vi "VoltageScan_easy.vi"() -> ()   [LabVIEW 2016]
uses:
  Input_parameters.ctl
  Dynamic_data.ctl
panel:
  out "Single channel":cluster{"X":dbl[], "Y":dbl[]}[](graph) caption="XY Graph"
  out "Voltages":cluster{"X":dbl[], "Y":dbl[]}[](graph) caption="XY Graph"
  out "Channels":cluster{i32[], dbl[]}[](graph) caption="XY Graph"
  out "Current channel":dbl format="%#_13g"
  out "Current voltage (V)":dbl format="%#_13g"
  in  "Stop":bool
  in  "Input parameters":T1={"Measurement type"=enum."Test", "Sensor type"=enum."One channel", "Input file"="", "Output file"="test.txt", "Open after execution?"=FALSE, "Display channel"=0, "Voltage Delay (s)"=0.5, "Switch Delay (s)"=0.01, "VISA resource name source"="", "VISA resource name LCR"="", "Voltage Limit (V)"=1000.0, "Enable Voltage Auto Range (T:Enable)"=TRUE, "Voltage Manual Range (1.0)"=1.0, "Compliance  Level (uA)"=10.0} {"Voltage Limit (V)" format="%#_13g"; "Voltage Delay (s)" format="%#_13g"; "Switch Delay (s)" format="%#_13g"}
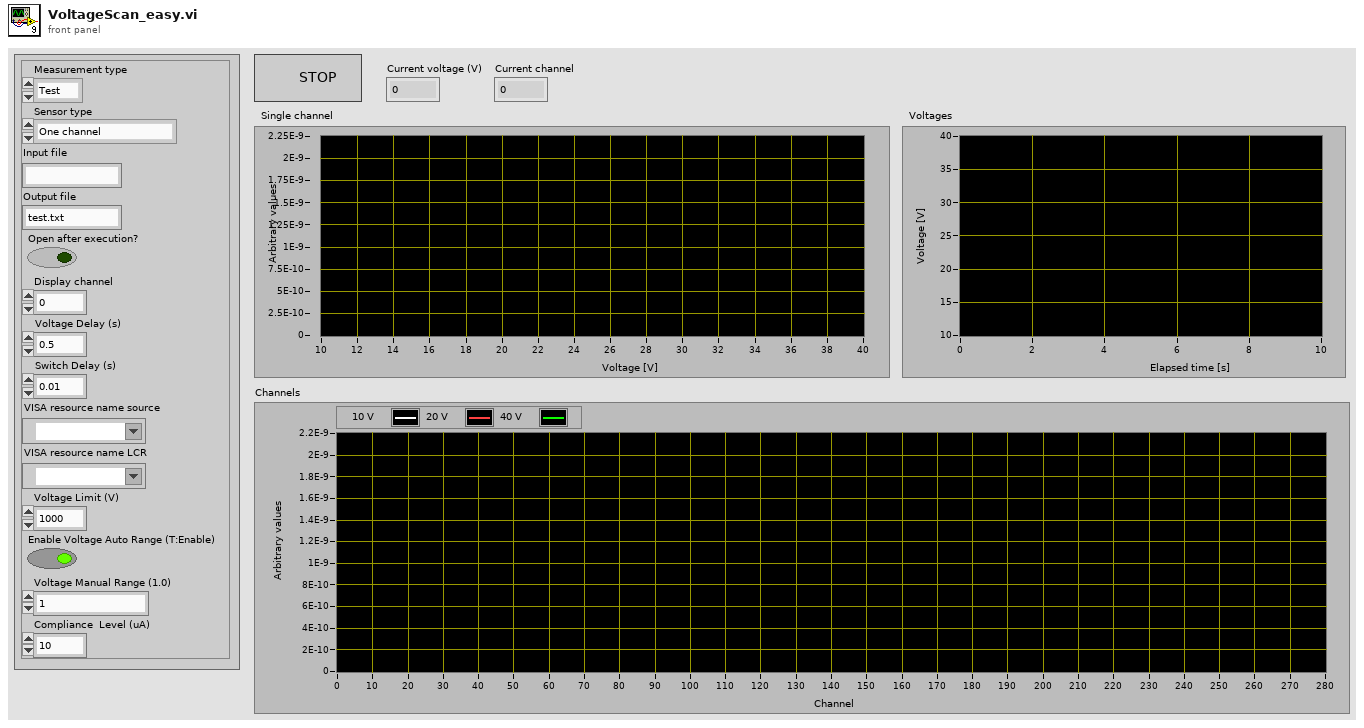
[diagram p1: front panel]
types:
  T1 = typedef "Input_parameters.ctl" = cluster{"Measurement type":enum16{"IV", "CV", "Test"}, "Sensor type":enum16{"6''", "8''", "One channel"}, "Input file":string, "Output file":string, "Open after execution?":bool, "Display channel":i32, "Voltage Delay (s)":dbl, "Switch Delay (s)":dbl, "VISA resource name source":refnum<visa-resource-name>, "VISA resource name LCR":refnum<visa-resource-name>, "Voltage Limit (V)":dbl, "Enable Voltage Auto Range (T:Enable)":bool, "Voltage Manual Range (1.0)":dbl, "Compliance  Level (uA)":dbl}
  T2 = typedef "Dynamic_data.ctl" = cluster{"Input file":path, "Output file":path, "Y-label text":string, "Voltage array":dbl[][], "Current set voltage":dbl, "Voltage column":dbl[], "Pad number column":dbl[], "Data  column":dbl[], "Number of voltages":i32, "Compliance current (A)":dbl}
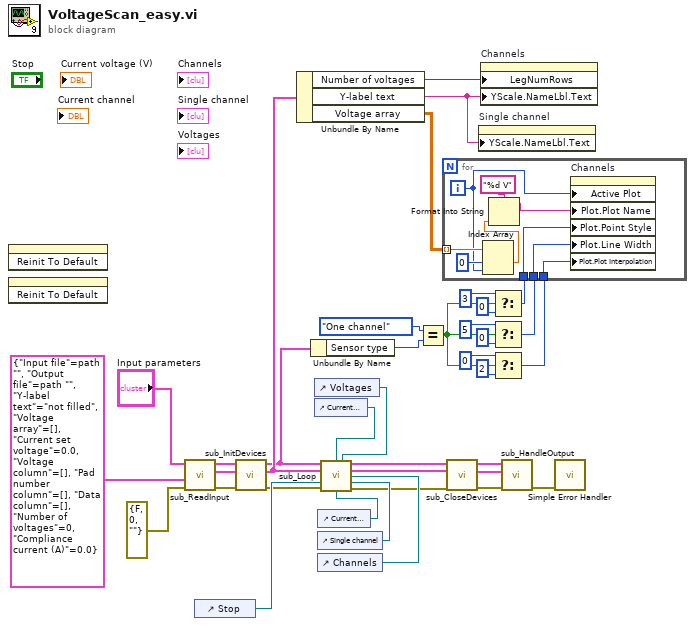
[diagram p0: block diagram]
diagram:
  n1 = invoke on="Stop" class="Bool (strict)" method="Reinit To Default"() -> ()  [unwired: 3 in, 3 out]
  n2 = invoke on="Single channel" class="XYGraph (strict)" method="Reinit To Default"() -> ()  [unwired: 3 in, 3 out]
  n3 = call "sub_ReadInput.vi"("error in (no error)"=errorcluster {"status"=FALSE, "code"=0, "source"=""}, "Dynamic data"=T2 {"Input file"=path "", "Output file"=path "", "Y-label text"="not filled", "Voltage array"=[], "Current set voltage"=0.0, "Voltage column"=[], "Pad number column"=[], "Data  column"=[], "Number of voltages"=0, "Compliance current (A)"=0.0}, "Input parameters"="Input parameters") -> ("error out"=w34:errorcluster, "Dynamic data"=w29:T2, "Input parameters"=w35:T1)  [unwired: 6 in]
  n4 = control-ref of="Stop"() -> (w25:refnum<vi>)
  n5 = call "sub_InitDevices.vi"("error in (no error)"=w34, "Dynamic data"=w29, "Input parameters"=w35) -> ("error out"=w24:errorcluster, "Dynamic data"=w26:T2, "Input parameters"=w6:T1)  [unwired: 6 in]
  n6 = Unbundle By Name(w26) -> ("Number of voltages"=w27:i32, "Y-label text"=w15:string, "Voltage array"=w1:dbl[][])
  n7 = Unbundle By Name(w6) -> ("Sensor type"=w5:enum16{"6''", "8''", "One channel"})
  n8 = control-ref of="Voltages"() -> (w16:refnum<vi>)
  n9 = control-ref of="Current voltage (V)"() -> (w18:refnum<vi>)
  n10 = control-ref of="Current channel"() -> (w17:refnum<vi>)
  n11 = control-ref of="Single channel"() -> (w20:refnum<vi>)
  n12 = control-ref of="Channels"() -> (w21:refnum<vi>)
  n13 = call "sub_Loop.vi"("Input parameters"=w6, "Current voltage"=w18, "Voltages"=w16, "Dynamic data 2"=w26, "Channels"=w21, "Stop"=w25, "Single channel"=w20, "error in (no error)"=w24, "Current channel"=w17) -> ("Input parameters"=w23:T1, "Dynamic data"=w22:T2, "error out"=w19:errorcluster)  [unwired: 4 in]
  n14 = Equal?(x=enum16{"6''", "8''", "One channel"}."One channel" ("Sensor type 2"), y=w5) -> (x = y?=w7:bool)
  n15 = call "sub_CloseDevices.vi"("error in (no error)"=w19, "Dynamic data 2"=w22, "Input parameters"=w23) -> ("error out"=w33:errorcluster, "Dynamic data"=w28:T2, "Input parameters"=w32:T1)  [unwired: 6 in]
  n16 = property on="Single channel" class="XYGraph (strict)"("YScale.NameLbl.Text"=w15) -> ()  [unwired: 2 in, 2 out]
  n17 = property on="Channels" class="XYGraph (strict)"("LegNumRows"=w27, "YScale.NameLbl.Text"=w15) -> ()  [unwired: 2 in, 2 out]
  n18 = Select(t=u8 3 ("Plot.Point Style"), s=w7, f=u8 0 ("Plot.Point Style")) -> (s? t:f=w2:u8)
  n19 = Select(t=u8 5 ("Plot.Point Style"), s=w7, f=u8 0 ("Plot.Point Style")) -> (s? t:f=w3:u8)
  n20 = Select(t=u8 0 ("Plot.Point Style"), s=w7, f=u8 2 ("Plot.Point Style")) -> (s? t:f=w4:u8)
  n21 = for {
    tunnel: w4 -> [w45]
    tunnel: w3 -> [w44]
    tunnel: w2 -> [w43]
    tunnel: w1 -> [w42] mode=indexing
    i -> [w38]
    n22 = Index Array(array=w42, index #1=0 ("index"), index #2=w38) -> (element #1=w40:dbl)  [unwired: 1 out]
    n23 = Format Into String(format string="%d V", w40) -> (resulting string=w46:string)  [unwired: 2 in, 1 out]
    n24 = property on="Channels" class="XYGraph (strict)"("Active Plot"=w38, "Plot.Plot Name"=w46, "Plot.Point Style"=w43, "Plot.Line Width"=w44, "Plot.Plot Interpolation"=w45) -> ()  [unwired: 2 in, 2 out]
  }
  n25 = call "sub_HandleOutput.vi"("error in (no error)"=w33, "Dynamic data 2"=w28, "Input parameters"=w32) -> ("error out"=w31:errorcluster)  [unwired: 6 in, 2 out]
  n26 = call <vilib>:"Simple Error Handler.vi"("error in (no error)"=w31) -> ()  [unwired: 4 in, 5 out]
